vi "save_data_order_log.vi"(7 "variable indices":u32[][](array[numeric]), 8 "error in (no error)":errorcluster, 9 "Variable Names Array":string[](array[string]), 11 "file path":path) -> (0 "error out":errorcluster)   [LabVIEW 2013]
uses:
  <vilib>/Utility/file.llb/Write To Spreadsheet File (string).vi
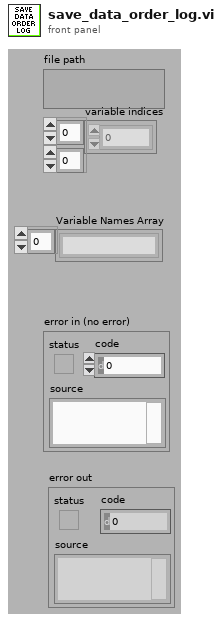
[diagram p1: front panel]
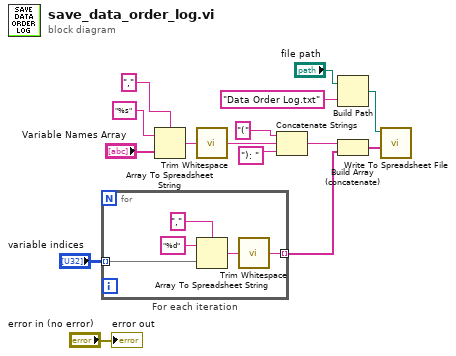
[diagram p0: block diagram]
diagram:
  n1 = for "For each iteration" {
    tunnel: "variable indices" -> [w20] mode=indexing
    tunnel: [w17] -> w2 mode=indexing
    n2 = Array To Spreadsheet String(delimiter (Tab)=",", array=w20, 3:"%d" ("format string")) -> (spreadsheet string=w16:string)
    n3 = call <vilib>:"Trim Whitespace.vi"("string"=w16) -> ("trimmed string"=w17:string)  [unwired: 1 in]
  }
  n4 = Array To Spreadsheet String(delimiter (Tab)=",", array="Variable Names Array", 3:"%s" ("format string")) -> (spreadsheet string=w11:string)
  n5 = call <vilib>:"Trim Whitespace.vi"("string"=w11) -> ("trimmed string"=w12:string)  [unwired: 1 in]
  n6 = Concatenate Strings("(" ("string"), w12, "): " ("string")) -> (w6:string)
  n7 = Build Path(base path="file path", name or relative path="Data Order Log.txt") -> (appended path=w13:path)
  n8 = Build Array (concatenate)(w6, w2) -> (w1:string[])
  n9 = call-poly <vilib>:"Write To Spreadsheet File.vi"("1D data"=w1, "file path (dialog if empty)"=w13) -> ()  [unwired: 6 in, 1 out]
  "error out" <- "error in (no error)"
